vi "FGV_Image.vi"(10 "Image_Cluster_in":T1={"Detector_info"={"No. of detectors"=0.0, "Detector_Array"=[], "Detector_Array_Numeric"=[]}, "Corner_info"={"Corner_Array"=[]}, "ROI"={"Corners"=[], "Detectors"=[]}, "Shape_Detect"={"Match_score"=0.0, "Curve Parameters"={"Extraction Mode"=0, "Edge Threshold"=75, "Edge Filter Size"=1, "Min Length"=25, "Row Search Step Size"=15, "Col Search Step Size"=15, "Max Endpoint Gap"=10, "Closed"=FALSE, "Subpixel"=FALSE}, "Match Options"={"Rotation"=FALSE, "Scale"=FALSE, "Occlusion"=FALSE, "Range Settings"=[]}, "Circle Descriptor"={"Min Radius"=3.0, "Max Radius"=500.0}}, "Path"={"Config"=path "", "Map"=path ""}, "Map"={"X_resolution"=0, "Y_resolution"=0, "Image"=refnum}, "Conversion_factor"=0.0} {"Shape_Detect"."Match Options"."Range Settings"."Match Constraints" items=["Rotation Angle (degrees)", "Scale Factor (%)", "Occlusion (%)"]; "Shape_Detect"."Curve Parameters"."Max Endpoint Gap" min=0; "Shape_Detect"."Curve Parameters"."Col Search Step Size" min=1 max=255 step=1; "Shape_Detect"."Curve Parameters"."Row Search Step Size" min=1 max=255 step=1; "Shape_Detect"."Curve Parameters"."Min Length" min=0; "Shape_Detect"."Curve Parameters"."Edge Filter Size" items=["Fine", "Normal", "Controur Tracing"]; "Shape_Detect"."Curve Parameters"."Edge Threshold" min=1 max=65535 step=1; "Shape_Detect"."Curve Parameters"."Extraction Mode" items=["Normal", "Uniform Regions"]; "ROI"."Detectors"."Contours"."Type" items=["No Selection", "Point", "Line", "Rectangle", "Oval", "Polygon", "Freehand Region", "Annulus", "Unused2", "Unused3", "Broken Line", "Freehand Line", "Rotated Rectangle"]; "ROI"."Corners"."Contours"."Type" items=["No Selection", "Point", "Line", "Rectangle", "Oval", "Polygon", "Freehand Region", "Annulus", "Unused2", "Unused3", "Broken Line", "Freehand Line", "Rotated Rectangle"]}, 11 "Action":enum16{"Read", "Write", ""}(ring)) -> (2 "Image_Cluster_out":T1={"Detector_info"={"No. of detectors"=0.0, "Detector_Array"=[], "Detector_Array_Numeric"=[]}, "Corner_info"={"Corner_Array"=[]}, "ROI"={"Corners"=[], "Detectors"=[]}, "Shape_Detect"={"Match_score"=0.0, "Curve Parameters"={"Extraction Mode"=0, "Edge Threshold"=75, "Edge Filter Size"=1, "Min Length"=25, "Row Search Step Size"=15, "Col Search Step Size"=15, "Max Endpoint Gap"=10, "Closed"=FALSE, "Subpixel"=FALSE}, "Match Options"={"Rotation"=FALSE, "Scale"=FALSE, "Occlusion"=FALSE, "Range Settings"=[]}, "Circle Descriptor"={"Min Radius"=3.0, "Max Radius"=500.0}}, "Path"={"Config"=path "", "Map"=path ""}, "Map"={"X_resolution"=0, "Y_resolution"=0, "Image"=refnum}, "Conversion_factor"=0.0} {"Shape_Detect"."Match Options"."Range Settings"."Match Constraints" items=["Rotation Angle (degrees)", "Scale Factor (%)", "Occlusion (%)"]; "Shape_Detect"."Curve Parameters"."Max Endpoint Gap" min=0; "Shape_Detect"."Curve Parameters"."Col Search Step Size" min=1 max=255 step=1; "Shape_Detect"."Curve Parameters"."Row Search Step Size" min=1 max=255 step=1; "Shape_Detect"."Curve Parameters"."Min Length" min=0; "Shape_Detect"."Curve Parameters"."Edge Filter Size" items=["Fine", "Normal", "Controur Tracing"]; "Shape_Detect"."Curve Parameters"."Edge Threshold" min=1 max=65535 step=1; "Shape_Detect"."Curve Parameters"."Extraction Mode" items=["Normal", "Uniform Regions"]; "ROI"."Detectors"."Contours"."Type" items=["No Selection", "Point", "Line", "Rectangle", "Oval", "Polygon", "Freehand Region", "Annulus", "Unused2", "Unused3", "Broken Line", "Freehand Line", "Rotated Rectangle"]; "ROI"."Corners"."Contours"."Type" items=["No Selection", "Point", "Line", "Rectangle", "Oval", "Polygon", "Freehand Region", "Annulus", "Unused2", "Unused3", "Broken Line", "Freehand Line", "Rotated Rectangle"]})   [LabVIEW 2020]
uses:
  Controls/Image_Cluster.ctl
  <vilib>/vision/Pattern Matching.llb/IMAQ Curve Parameters.ctl
  <vilib>/vision/Shape Detection.llb/ShapeDetectionMatchOptions.ctl
  <vilib>/vision/Pattern Matching.llb/IMAQ Match Range Setting.ctl
panel:
  # "detector array columns\n0 - name\n1 - S for shelf, R for reading area, SM for segragation machine\n2 - X_UL\n3 - Y_UL\n4- X_LR\n5 - Y_LR\n6 - detection_radius \n7 - center coordinate X\n8 - center coordinate Y\n9 - found? (0 or 1) \n10 - distance from book coordinates\n\n\nafter detection of the circles, the detector_array should be modified to delete all \ndetectors that were not found in the map\n-kasi after magdetect, magdidistance formula tayo from all centers\nto the given coordinate, and wala naman tayong distance formula na magagawa kapag \nhindi detected ang circle"
  # "Corner array columns\n0 - center coordinate X\n1 - center coordinate Y\n2 - found? (1 or 0)"
  # "Range"
  # "Range"
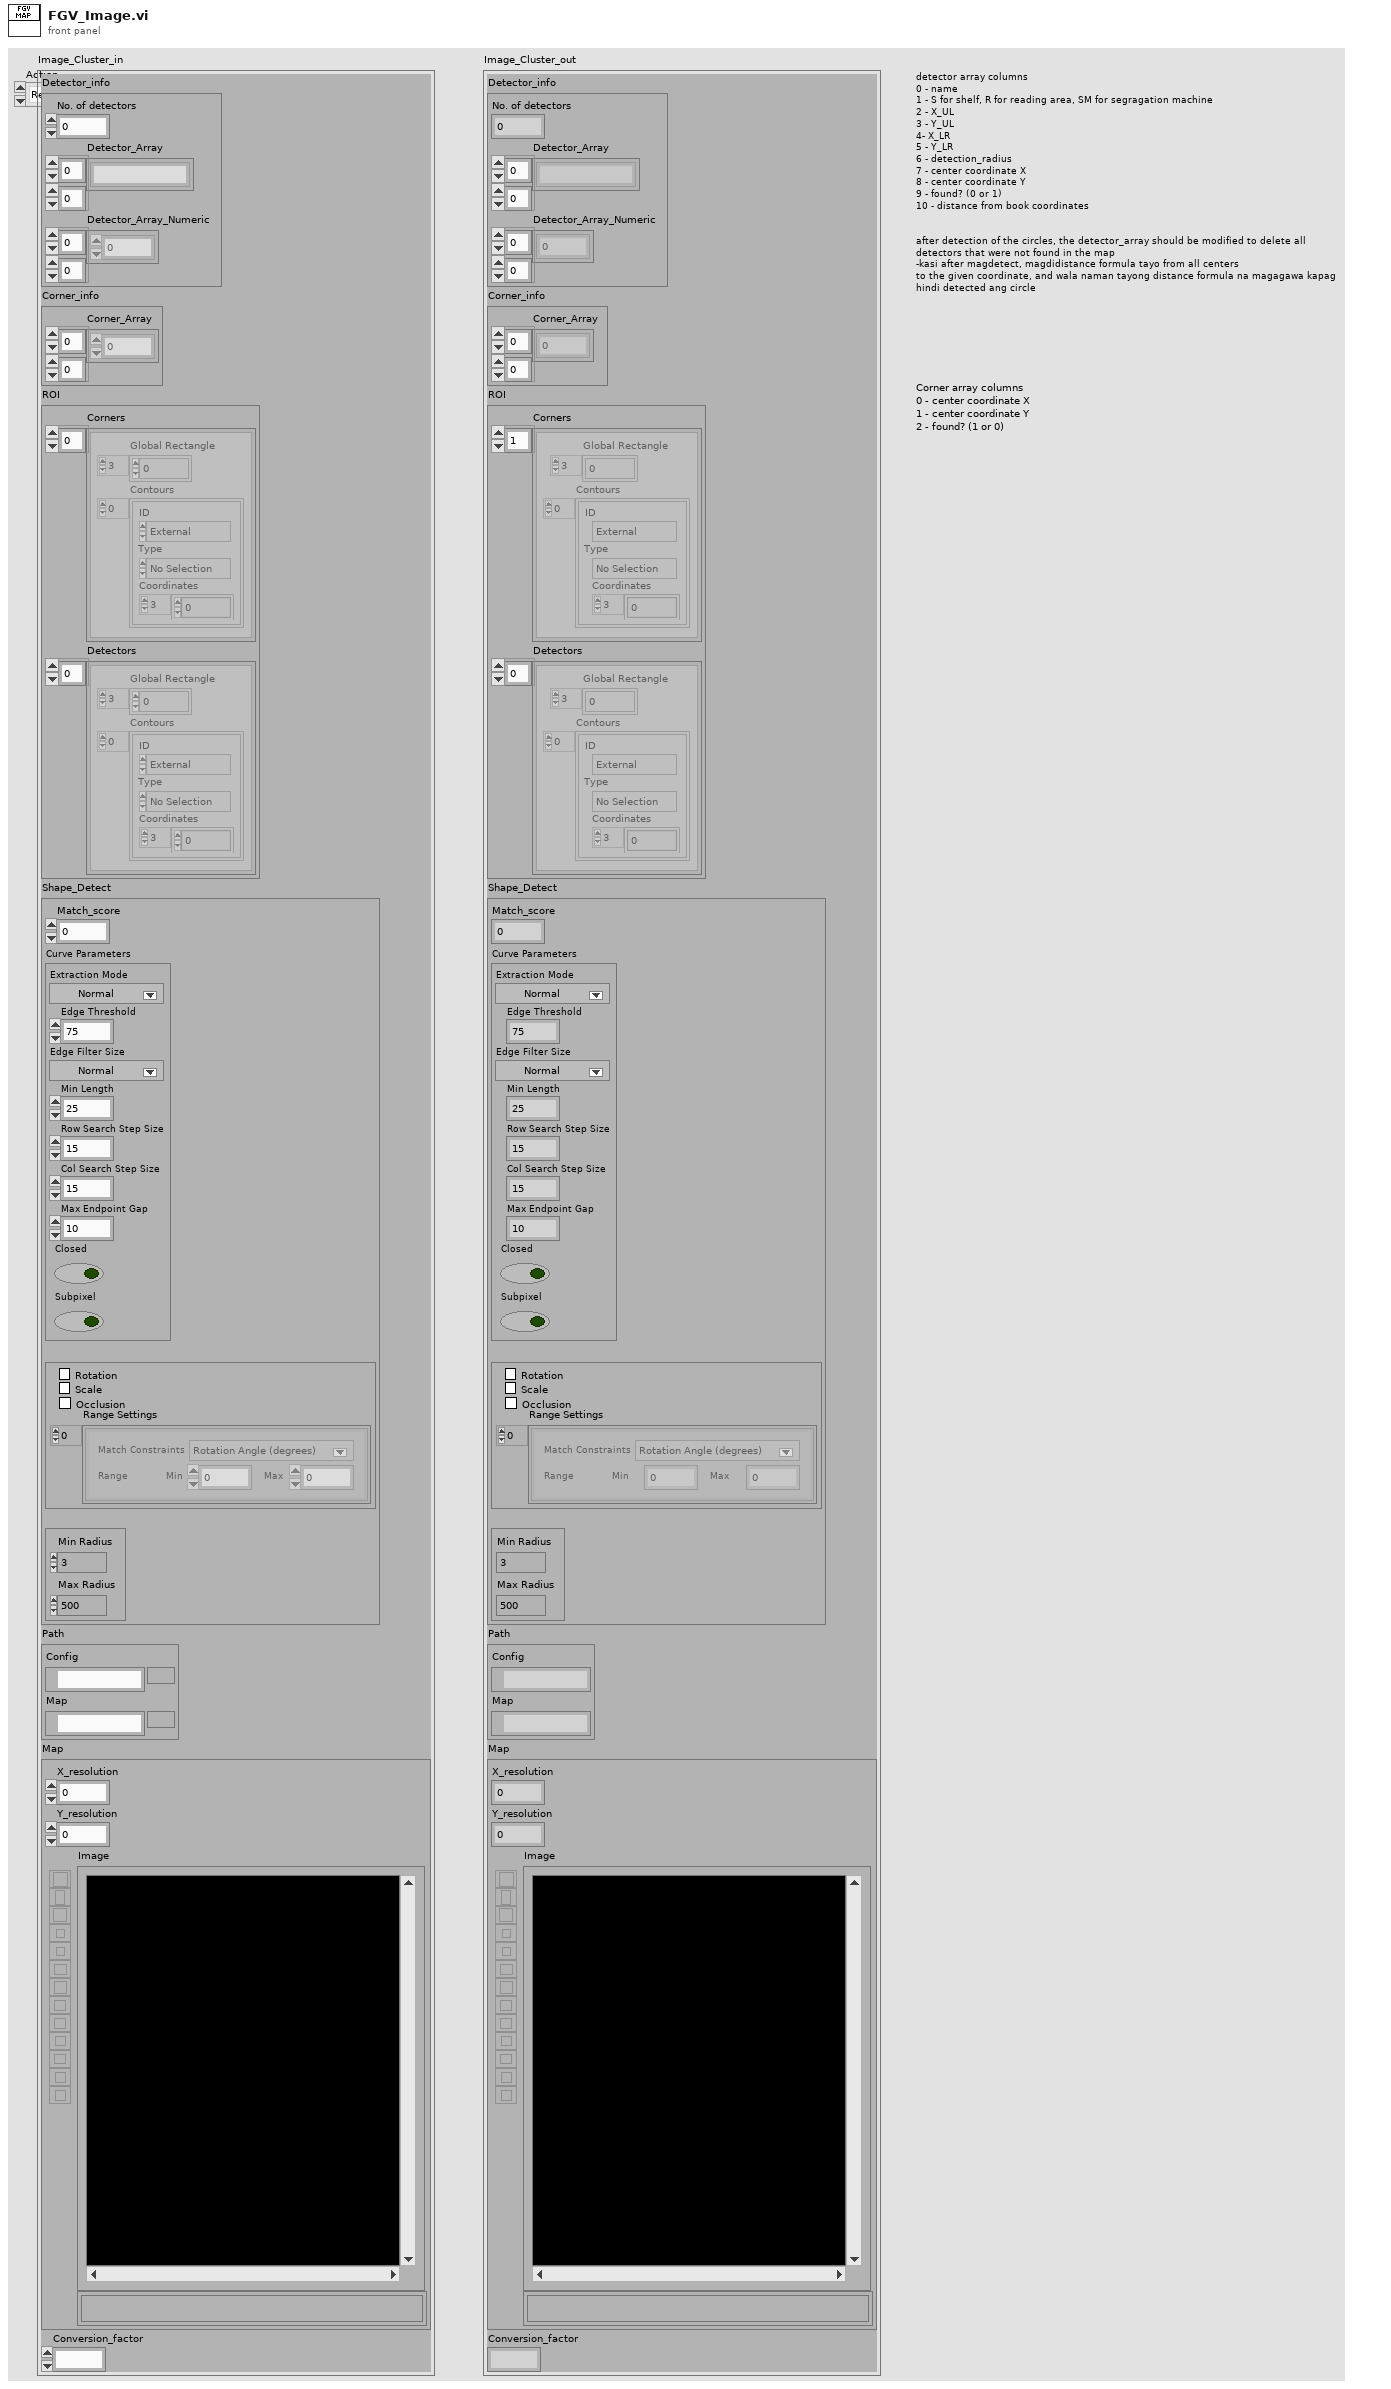
[diagram p1: front panel]
types:
  T1 = typedef "Image_Cluster.ctl" = cluster{"Detector_info":cluster{"No. of detectors":dbl, "Detector_Array":string[][], "Detector_Array_Numeric":dbl[][]}, "Corner_info":cluster{"Corner_Array":dbl[][]}, "ROI":cluster{"Corners":cluster{"Global Rectangle":i32[], "Contours":cluster{"ID":enum32{"External", "Internal"}, "Type":u32, "Coordinates":i32[]}[]}[], "Detectors":cluster{"Global Rectangle":i32[], "Contours":cluster{"ID":enum32{"External", "Internal"}, "Type":u32, "Coordinates":i32[]}[]}[]}, "Shape_Detect":cluster{"Match_score":dbl, "Curve Parameters":T2, "Match Options":T3, "Circle Descriptor":cluster{"Min Radius":dbl, "Max Radius":dbl}}, "Path":cluster{"Config":path, "Map":path}, "Map":cluster{"X_resolution":i32, "Y_resolution":i32, "Image":T5}, "Conversion_factor":dbl}
  T2 = typedef "IMAQ Curve Parameters.ctl" = cluster{"Extraction Mode":u32, "Edge Threshold":i32, "Edge Filter Size":u32, "Min Length":i32, "Row Search Step Size":i32, "Col Search Step Size":i32, "Max Endpoint Gap":i32, "Closed":bool, "Subpixel":bool}
  T3 = typedef "ShapeDetectionMatchOptions.ctl" = cluster{"Rotation":bool, "Scale":bool, "Occlusion":bool, "Range Settings":T4[]}
  T4 = typedef "IMAQ Match Range Setting.ctl" = cluster{"Match Constraints":u32, "Min":dbl, "Max":dbl}
  T5 = typedef "IMAQ Image.ctl" = refnum<image>
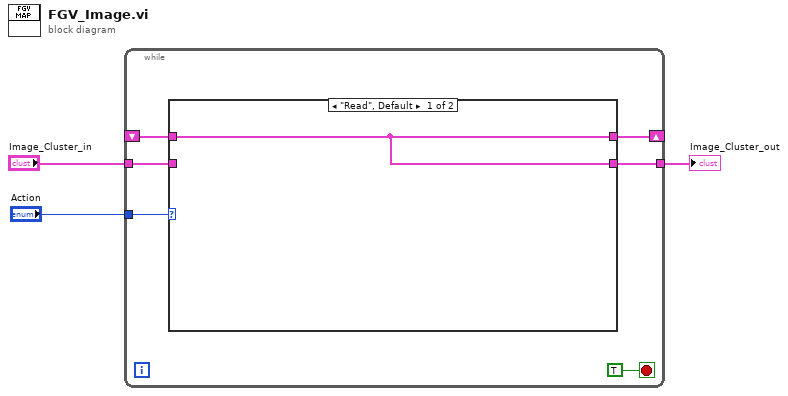
[diagram p0: block diagram]
diagram:
  n1 = while {
    tunnel: "Action" -> [w8]
    shift-right: [w4] -> _
    shift-left: _ -> [w5]
    tunnel: "Image_Cluster_in" -> [w7]
    tunnel: [w6] -> w1
    stop <- TRUE stop-if-true
    n2 = case shown="\"Read\", Default" w8 {
      tunnel: w7 -> [_ w11]
      tunnel: [w10 w11] -> w6
      tunnel: w5 -> [w10 _]
      tunnel: [w10 w11] -> w4
      frame "Read", Default {
      }
      frame "Write" {
      }
    }
  }
  "Image_Cluster_out" <- w1
